vi "Evaluate Self Test BIST.vi"(1 "String In":string) -> (0 "Test OK":bool)   [LabVIEW 2022 SP3]
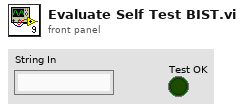
[diagram p1: front panel]
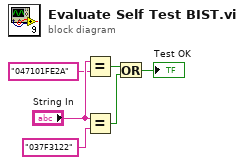
[diagram p0: block diagram]
diagram:
  n1 = Equal?(x="String In", y="047101FE2A") -> (x = y?=w5:bool)
  n2 = Equal?(x="String In", y="037F3122" ("Self Test BIST")) -> (x = y?=w2:bool)
  n3 = Or(x=w5, y=w2) -> (x .or. y?=→"Test OK":bool)
